vi "Inputs.vi"(8 "error in (no error)":errorcluster, 11 "State in":T1={"State"=enum."Idle", "Start Time"=timestamp(0 s since 1904-01-01), "Configuration"={"Cycle Period"=0.0, "Mettler"={"VISA resource name"="", "Simulated?"=FALSE}, "Scale Type"=""}, "Current Time"=timestamp(0 s since 1904-01-01), "First Iteration"=FALSE, "Data"={"Scale Read(g)"=0.0}, "Process Name"="", "Log Started"=FALSE}) -> (0 "error out":errorcluster, 3 "State out":T1={"State"=enum."Idle", "Start Time"=timestamp(0 s since 1904-01-01), "Configuration"={"Cycle Period"=0.0, "Mettler"={"VISA resource name"="", "Simulated?"=FALSE}, "Scale Type"=""}, "Current Time"=timestamp(0 s since 1904-01-01), "First Iteration"=FALSE, "Data"={"Scale Read(g)"=0.0}, "Process Name"="", "Log Started"=FALSE})   [LabVIEW 2021, in "Scale Module.lvlib" / "Scale Module Engine.lvlib"]
uses:
  Scale Module Engine.lvlib
  State Cluster.ctl
  State Enum.ctl
  Feed Module/Controls/Scale Module Settings Cluster.ctl
  Mettler Toledo/Controls/Settings Cluster.ctl
  Tag VIs/Tag FGV Operation Enum.ctl
  Mettler Toledo/Mettler Toledo.lvlib
  Shared Variables/Dynamic Shared Variables.lvlib
  Scale Module.lvlib
panel:
  # "Scale Settings"
  # "Scale Settings"
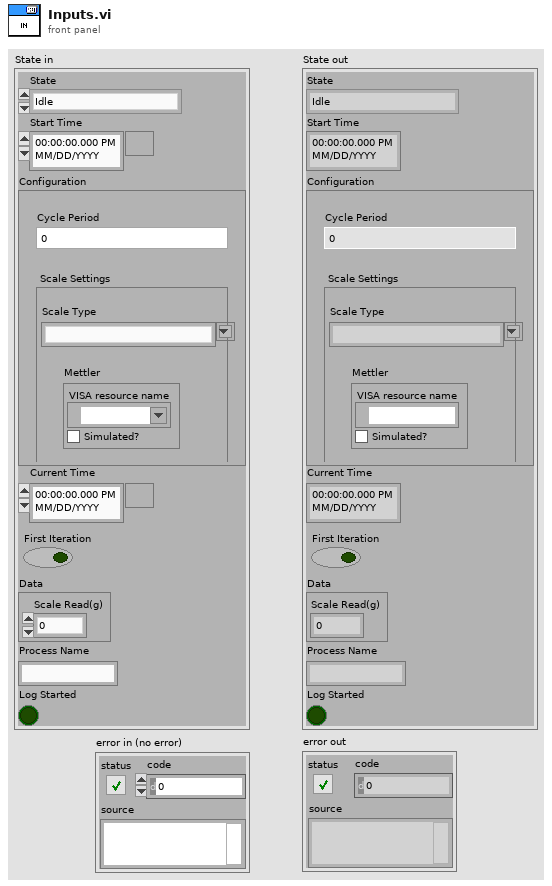
[diagram p1: front panel]
types:
  T1 = typedef "Scale Module.lvlib/Scale Module Engine.lvlib/State Cluster.ctl" = cluster{"State":T2, "Start Time":timestamp, "Configuration":T3, "Current Time":timestamp, "First Iteration":bool, "Data":cluster{"Scale Read(g)":dbl}, "Process Name":string, "Log Started":bool}
  T2 = typedef "Scale Module.lvlib/Scale Module Engine.lvlib/State Enum.ctl" = enum16{"Measuring", "Idle"}
  T3 = typedef "Scale Module.lvlib/Scale Module Settings Cluster.ctl" = cluster{"Cycle Period":dbl, "Mettler":T4, "Scale Type":string}
  T4 = typedef "Mettler Toledo.lvlib/Settings Cluster.ctl" = cluster{"VISA resource name":refnum<visa-resource-name>, "Simulated?":bool}
  T5 = typedef "Tag FGV Operation Enum.ctl" = enum16{"Init", "Set Notification Queue", "Create Tag", "Commit", "Write Tag (Numeric)", "Write Tag (Boolean)", "Read All Tags", "Read One Tag", "Delete Tag Category", "Set Alarm Parameters (Numeric)", "Set Alarm Parameters (Boolean)", "Enable All Alarms", "Disable All Alarms", "Delete All Tags", "Read Alarms", "Ack Alarm", "Read Alarm Parameters (Numeric)", "Read Alarm Parameters (Boolean)"}
  T6 = cluster{"Scale Tag":string, "Output Device Tag":string}
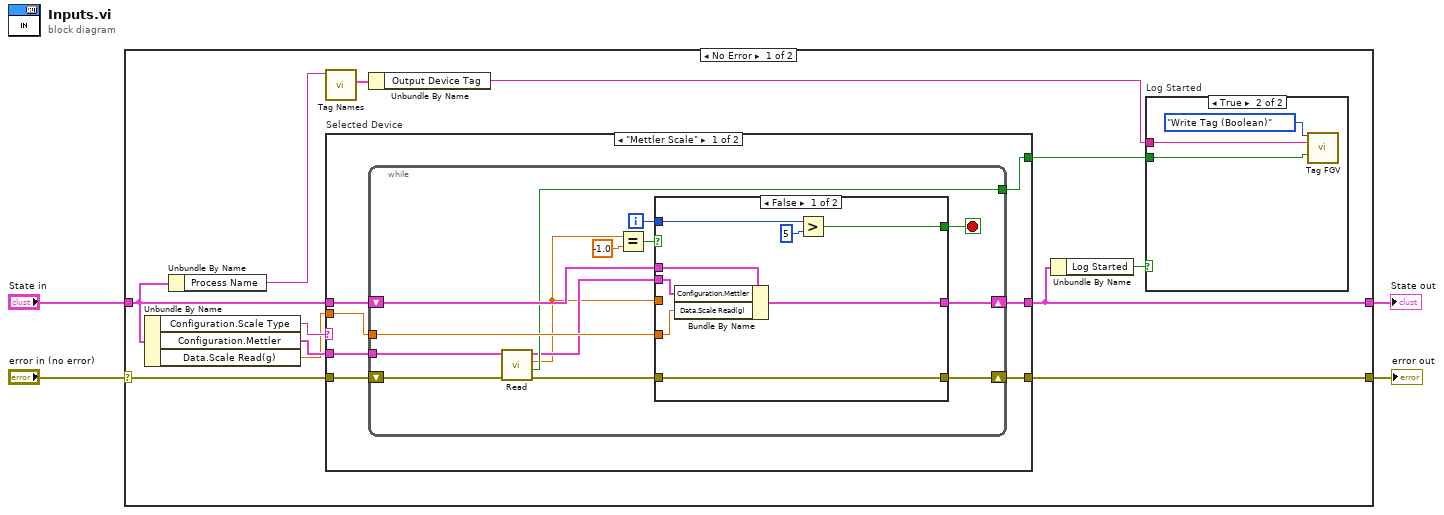
[diagram p0: block diagram]
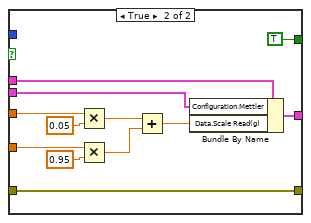
[diagram p3: hidden frame]
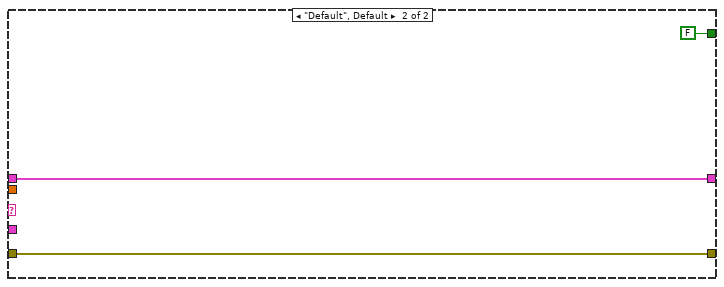
[diagram p4: hidden frame]
diagram:
  n1 = case shown="No Error" "error in (no error)" {
    selector: "error in (no error)" -> [w14 w65]
    tunnel: [w13 w65] -> w1
    tunnel: "State in" -> [w10 w64]
    tunnel: [w6 w64] -> w2
    frame No Error {
      n2 = Unbundle By Name(w10) -> ("Configuration.Scale Type"=w16:string, "Configuration.Mettler"=w15:T4, "Data.Scale Read(g)"=w12:dbl)
      n3 = Unbundle By Name(w10) -> ("Process Name"=w9:string)
      n4 = call "Tag Names.vi"("Process Name"=w9) -> ("Scale Tags"=w8:T6)  [unwired: 8 in, 2 out]
      n5 = case "Selected Device" shown="\"Mettler Scale\"" w16 {
        tunnel: w10 -> [w24 w63]
        tunnel: [w23 w63] -> w6
        tunnel: w15 -> [w25 _]
        tunnel: w14 -> [w26 w62]
        tunnel: [w22 w62] -> w13
        tunnel: w12 -> [w21 _]
        tunnel: [w20 FALSE ("Connection Error")] -> w11
        frame "Mettler Scale" {
          n6 = while {
            tunnel: w25 -> [w39]
            tunnel: w21 -> [w36]
            tunnel: [w35] -> w20
            shift-right: [w29] -> w22
            shift-left: w26 -> [w40]
            shift-right: [w37] -> w23
            shift-left: w24 -> [w38]
            i -> [w27]
            stop <- w30 stop-if-true
            n7 = call "Read.vi"("error in (no error)"=w40, "Mettler Settings in"=w39) -> ("error out"=w28:errorcluster, "Connection Error"=w35:bool, "mass (g)"=w32:dbl, "Mettler Settings out"=w34:T4)  [unwired: 6 in]
            n8 = Equal?(x=w32, y=-1.0) -> (x = y?=w31:bool)
            n9 = case shown="False" w31 {
              tunnel: w38 -> [w44 w60]
              tunnel: [w41 w59] -> w37
              tunnel: w36 -> [w42 w58]
              tunnel: w34 -> [w43 w57]
              tunnel: w32 -> [_ w56]
              tunnel: [w47 TRUE] -> w30
              tunnel: [w48 w49] -> w29
              tunnel: w28 -> [w48 w49]
              tunnel: w27 -> [w46 _]
              frame False {
                n10 = Bundle By Name(cluster=w44, "Configuration.Mettler"=w43, "Data.Scale Read(g)"=w42) -> (w41:T1)
                n11 = Greater?(x=w46, y=5) -> (0:w47:bool)
              }
              frame True {
                n12 = Multiply(x=w56, y=0.05) -> (x*y=w52:dbl)
                n13 = Multiply(x=w58, y=0.95) -> (x*y=w55:dbl)
                n14 = Add(x=w52, y=w55) -> (x+y=w51:dbl)
                n15 = Bundle By Name(cluster=w60, "Configuration.Mettler"=w57, "Data.Scale Read(g)"=w51) -> (w59:T1)
              }
            }
          }
        }
        frame "Default", Default {
        }
      }
      n16 = Unbundle By Name(w8) -> ("Output Device Tag"=w7:string)
      n17 = Unbundle By Name(w6) -> ("Log Started"=w5:bool)
      n18 = case "Log Started" shown="True" w5 {
        tunnel: w11 -> [_ w17]
        tunnel: w7 -> [_ w18]
        frame False {
        }
        frame True {
          n19 = call "Tag FGV.vi"("Operation"=Tag_FGV_Operation_Enum."Write Tag (Boolean)", "Tag Name"=w18, "Data"=w17) -> ()  [unwired: 5 in, 8 out]
        }
      }
    }
    frame Error {
    }
  }
  "error out" <- w1
  "State out" <- w2
